vi "SubsystemStatusToCAN.vi"(9 "NDashPage":u8, 11 "Subystem Status":T1) -> (3 "Array":u8[](array[numeric]))   [LabVIEW 2014]
uses:
  Vehicle Status/Subsystem Status.ctl
  Vehicle Status/Subsystem Status Severity.ctl
  Vehicle Status/Subsystem Status Message.ctl
  Global Data.vi
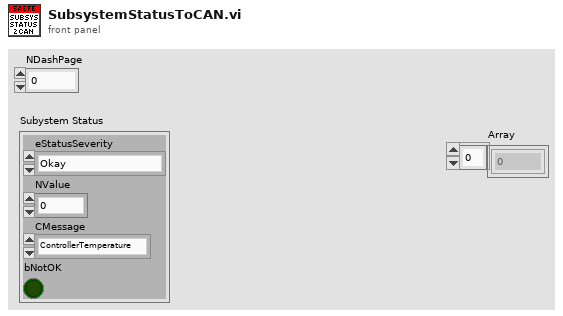
[diagram p1: front panel]
types:
  T1 = typedef "Subsystem Status.ctl" = cluster{"eStatusSeverity":T2, "NValue":sgl, "CMessage":T3, "bNotOK":bool}
  T2 = typedef "Subsystem Status Severity.ctl" = enum16{"Okay", "Short Warning", "Long Warning", "Return to Pits", "Error", "Danger"}
  T3 = typedef "Subsystem Status Message.ctl" = enum16{"ControllerTemperature", "MotorTemperature", "BatteryTemperature", "BatteryLowVoltage", "LVBattery", "sbRIOTemperature", "Precharge", "BSPD", "IMD", "RemoteReturnToPits", "EStopInterrupted", "NoCellComms", "MCOverSpeed", "MCOverCurrent", "MCOverVoltage", "MCInverterOverTemp", "MCDirectionCommand", "MCInverterTimeout", "MCDesatFault", "MCHWOverCurrent", "MCUnderVoltage", "MCCommandMessageLost", "MotorOverTemp", "MCModAOverTemp", "MCModBOverTemp", "MCModCOverTemp", "MCPCBOverTemp", "MCGateDrv1OverTemp", "MCDateDrv2OverTemp", "MCCurrentSensorFault", "MCResolverNotConnected", "ShutdownLatchTripped", "UnknownBMS", "RemoteEmergency"}
  T4 = typedef "SDashLEDs.ctl" = cluster{"bGreenLED":bool, "bYellowLED":bool, "bRedLED":bool}
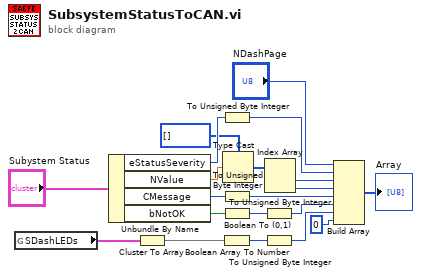
[diagram p0: block diagram]
diagram:
  n1 = global read "Global Data.vi" "SDashLEDs"() -> (w4:T4)
  n2 = Unbundle By Name("Subystem Status") -> ("eStatusSeverity"=w19:T2, "NValue"=w17:sgl, "CMessage"=w18:T3, "bNotOK"=w16:bool)
  n3 = Cluster To Array(cluster=w4) -> (array=w3:bool[])
  n4 = To Unsigned Byte Integer(number=w19) -> (unsigned 8bit integer=w12:u8)
  n5 = To Unsigned Byte Integer(number=w18) -> (unsigned 8bit integer=w9:u8)
  n6 = Boolean To (0,1)(Boolean=w16) -> (0, 1=w15:i16)
  n7 = Boolean Array To Number(Boolean array=w3) -> (number=w2:u32)
  n8 = Type Cast(type=u8[] [], x=w17) -> (*(type *) &x=w13:u8[])
  n9 = To Unsigned Byte Integer(number=w15) -> (unsigned 8bit integer=w8:u8)
  n10 = To Unsigned Byte Integer(number=w2) -> (unsigned 8bit integer=w1:u8)
  n11 = Index Array(array=w13) -> (element #1=w11:u8, element #2=w10:u8)  [unwired: 2 in]
  n12 = Build Array("NDashPage", w12, w11, w10, w9, w8, w1, u8 0 ("element")) -> (→"Array":u8[])
